vi "Demo - Read Digital Inputs.vi"() -> ()   [LabVIEW 2020]
uses:
  TypeDefs/Enum - Machine State.ctl
  <vilib>/ErrorRing/Error Ring.xnode
panel:
  out "Digital Inputs":bool[](array[boolean])
  in  "Stop":bool
  in  "DAQ IP Address":string="192.168.1.1"
  # "0     1     2     3     4     5     6     7     8     9    10   11   12   13   14   15"
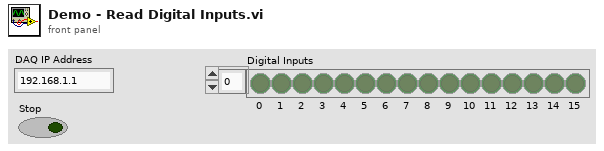
[diagram p1: front panel]
types:
  T1 = typedef "Enum - Machine State.ctl" = enum16{"Shutdown", "Start Streaming", "Initialize", "Read Streamed Data"}
  T2 = typedef "TypeDef - Cluster Representing Decoded JSON Message.ctl" = cluster{"timestamp":u64, "adc":cluster{"time":i32, "ch":i32, "data":i32}[], "dio":cluster{"time":i32, "mask":i32, "data":u16}[]}
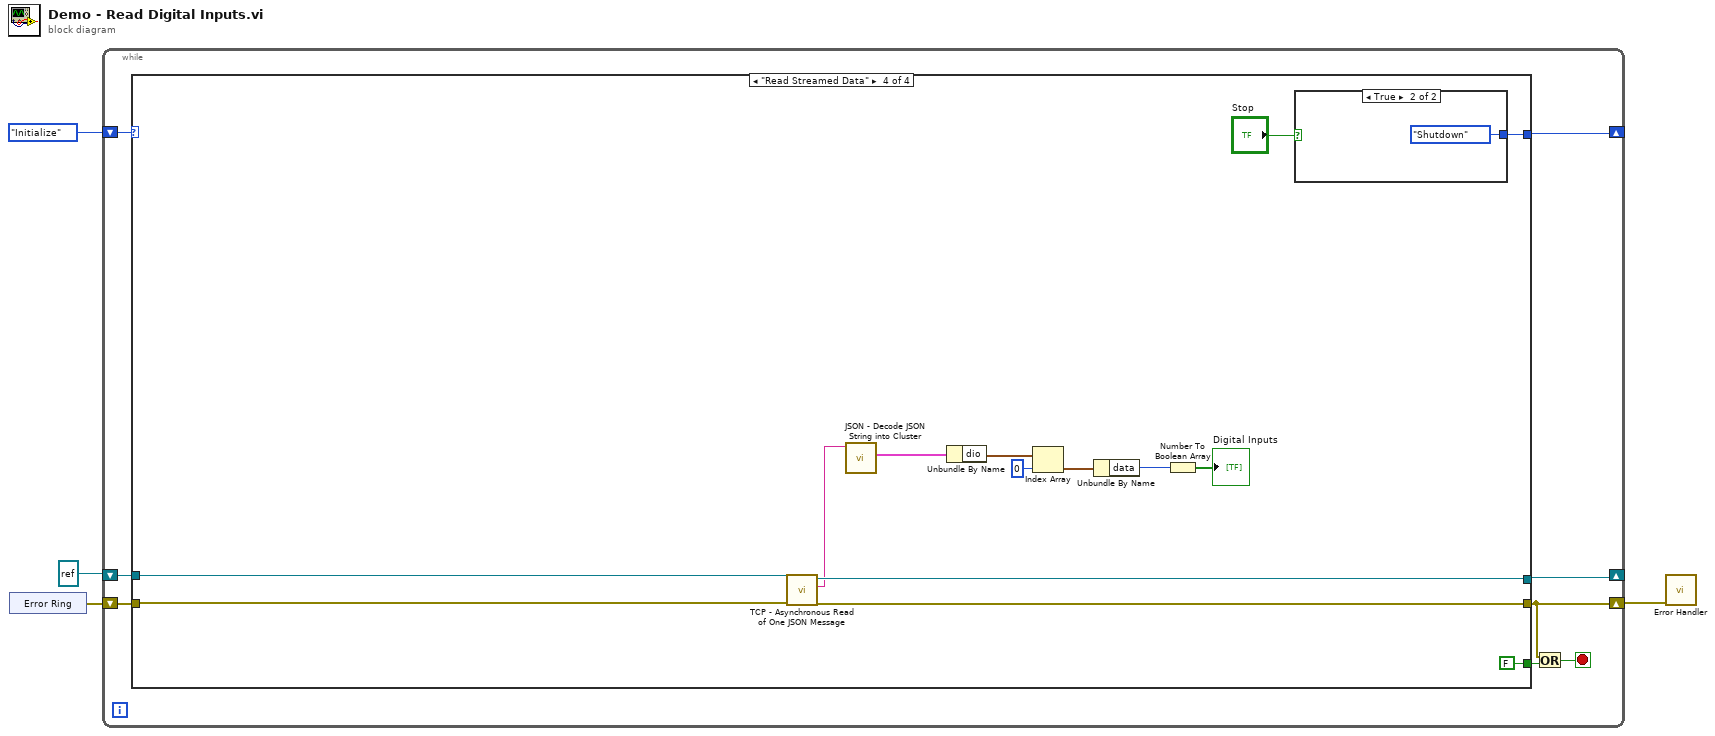
[diagram p0: block diagram]
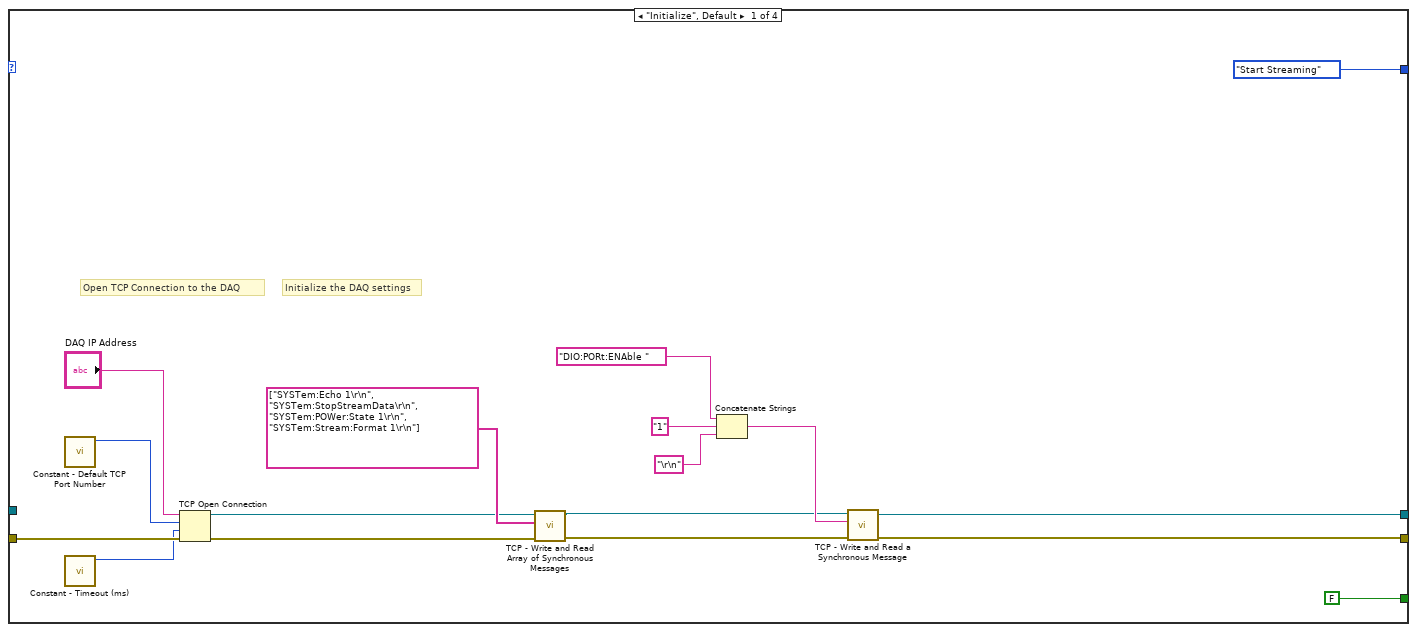
[diagram p2: hidden frame]
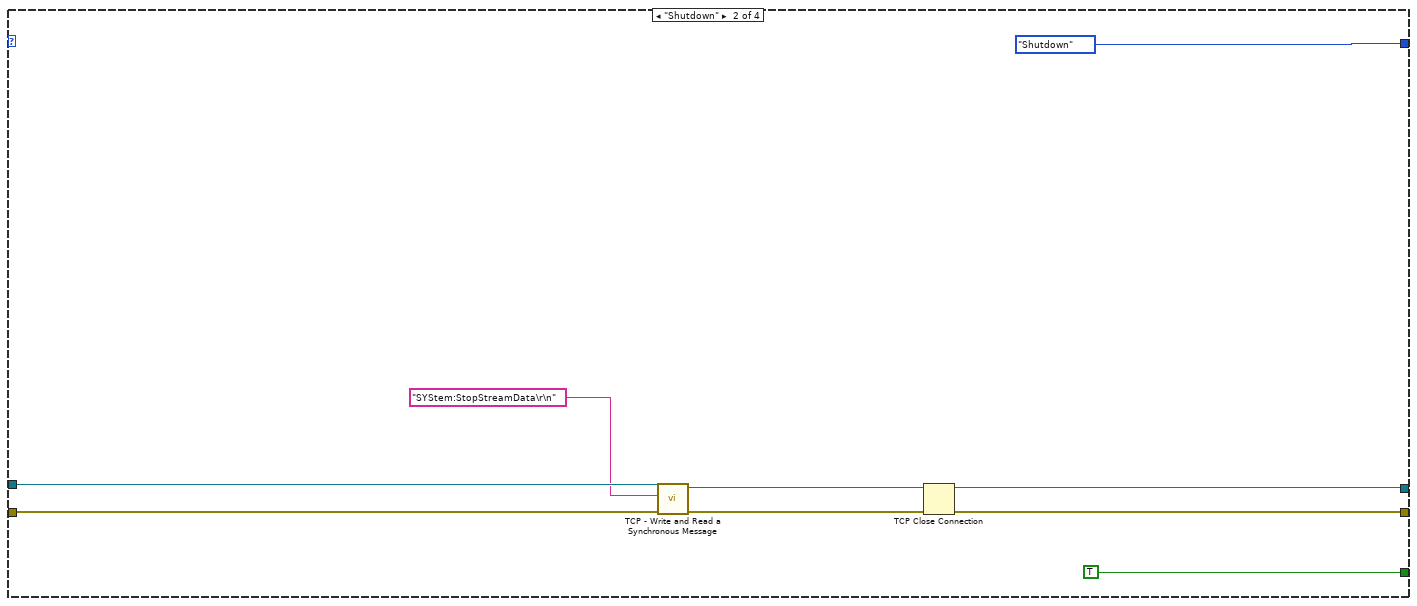
[diagram p3: hidden frame]
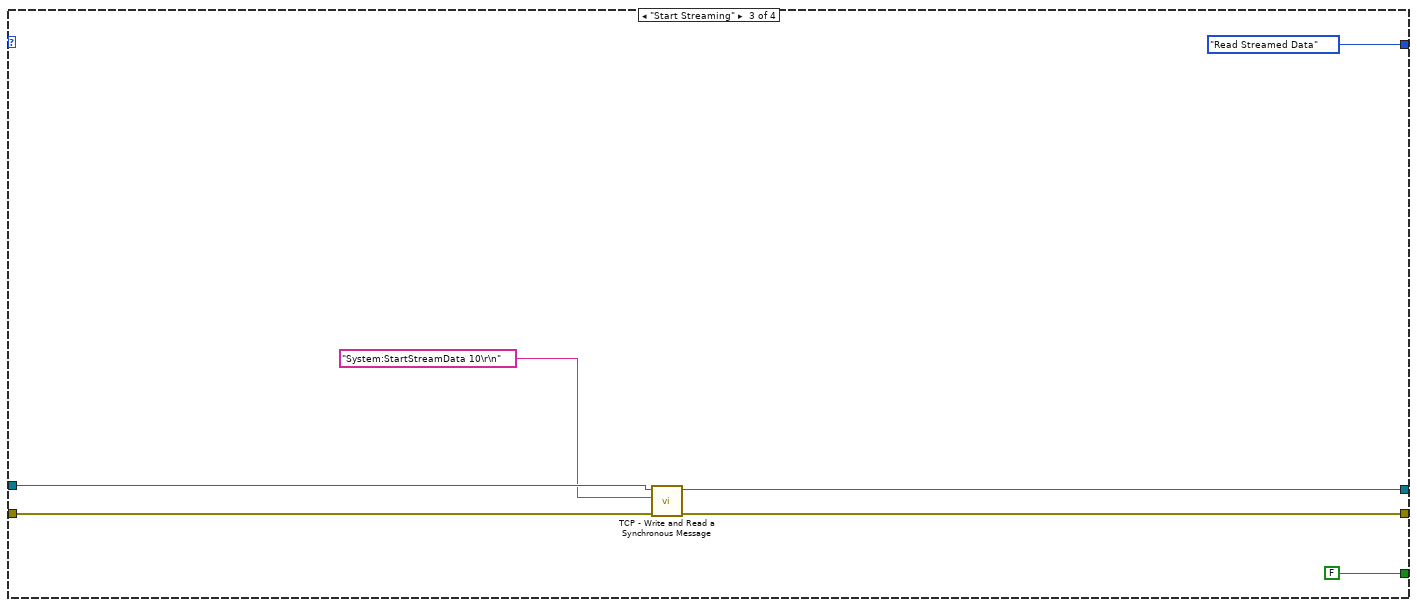
[diagram p4: hidden frame]
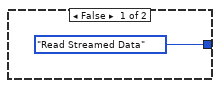
[diagram p5: hidden frame]
diagram:
  n1 = xnode "Error Ring"() -> ("error out"=w3:errorcluster)
  n2 = while {
    shift-right: [w6] -> w1
    shift-left: w3 -> [w11]
    shift-right: [w10] -> _
    shift-left: refnum<k5> refnum ("TCP Network Connection out") -> [w8]
    shift-right: [w9] -> _
    shift-left: Enum_-_Machine_State."Initialize" -> [w12]
    stop <- w5 stop-if-true
    n3 = case shown="\"Read Streamed Data\"" w12 {
      tunnel: w11 -> [w27 w35 w45 w55]
      tunnel: [w14 w30 w44 w56] -> w6
      tunnel: [w13 w31 w43 w57] -> w10
      tunnel: [Enum_-_Machine_State."Start Streaming" Enum_-_Machine_State."Shutdown" Enum_-_Machine_State."Read Streamed Data" w59] -> w9
      tunnel: [FALSE TRUE FALSE FALSE] -> w7
      tunnel: w8 -> [_ w36 w42 w58]
      frame "Initialize", Default {
        # "Open TCP Connection to the DAQ"
        # "Initialize the DAQ settings"
        n4 = call "Constant - Default TCP Port Number.vi"() -> ("Port"=w28:u16)  [unwired: 11 in]
        n5 = call "Constant - Timeout (ms).vi"() -> ("timeout (ms)"=w21:i32)  [unwired: 11 in]
        n6 = TCP Open Connection(address="DAQ IP Address", remote port or service name=w28, timeout ms (60000)=w21, error in (no error)=w27) -> (connection ID=w24:refnum<k5>, error out=w25:errorcluster)  [unwired: 1 in]
        n7 = call "TCP - Write and Read Array of Synchronous Messages.vi"("error in"=w25, "Array of Messages to Send"=string[] ["SYSTem:Echo 1\r\n", "SYSTem:StopStreamData\r\n", "SYSTem:POWer:State 1\r\n", "SYSTem:Stream:Format 1\r\n"], "TCP Network Connection in"=w24) -> ("error out"=w15:errorcluster, "TCP Network Connection out"=w16:refnum<k5>)  [unwired: 6 in, 1 out]
        n8 = Concatenate Strings("DIO:PORt:ENAble " ("Message to Send"), "1" ("string"), "\r\n" ("string")) -> (w18:string)
        n9 = call "TCP - Write and Read a Synchronous Message.vi"("error in"=w15, "Message to Send"=w18, "TCP Network Connection in"=w16) -> ("error out"=w14:errorcluster, "TCP Network Connection out"=w13:refnum<k5>)  [unwired: 6 in, 1 out]
      }
      frame "Shutdown" {
        n10 = call "TCP - Write and Read a Synchronous Message.vi"("error in"=w35, "Message to Send"="SYStem:StopStreamData\r\n", "TCP Network Connection in"=w36) -> ("error out"=w32:errorcluster, "TCP Network Connection out"=w33:refnum<k5>)  [unwired: 6 in, 1 out]
        n11 = TCP Close Connection(connection ID=w33, error in (no error)=w32) -> (connection ID out=w31:refnum<k5>, error out=w30:errorcluster)  [unwired: 1 in]
      }
      frame "Start Streaming" {
        n12 = call "TCP - Write and Read a Synchronous Message.vi"("error in"=w45, "Message to Send"="System:StartStreamData 10\r\n" ("data in"), "TCP Network Connection in"=w42) -> ("error out"=w44:errorcluster, "TCP Network Connection out"=w43:refnum<k5>)  [unwired: 6 in, 1 out]
      }
      frame "Read Streamed Data" {
        n13 = call "TCP - Asynchronous Read of One JSON Message.vi"("error in"=w55, "TCP Network Connection in"=w58) -> ("error out"=w56:errorcluster, "Received JSON Message"=w54:string, "TCP Network Connection out"=w57:refnum<k5>)  [unwired: 7 in]
        n14 = call "JSON - Decode JSON String into Cluster.vi"("JSON String"=w54) -> ("Data out"=w53:T2)  [unwired: 9 in, 1 out]
        n15 = Unbundle By Name(w53) -> ("dio"=w52:cluster{"time":i32, "mask":i32, "data":u16}[])
        n16 = Index Array(array=w52, index=0) -> (element=w50:cluster{"time":i32, "mask":i32, "data":u16})
        n17 = Unbundle By Name(w50) -> ("data"=w47:u16)
        n18 = Number To Boolean Array(number=w47) -> (Boolean array=→"Digital Inputs":bool[])
        n19 = case shown="True" "Stop" {
          tunnel: [Enum_-_Machine_State."Read Streamed Data" Enum_-_Machine_State."Shutdown"] -> w59
          frame False {
          }
          frame True {
          }
        }
      }
    }
    n20 = Or(x=w6, y=w7) -> (x .or. y?=w5:bool)
  }
  n21 = call "Error Handler.vi"("error in"=w1) -> ()  [unwired: 10 in, 1 out]
